vi "User Process Test.vi"() -> ()   [LabVIEW 2021, in "State Machine tests.lvlib"]
uses:
  State Machine tests.lvlib
  module/execution/State Machine runtime.lvclass
  module/execution/parameter user data.ctl
  module/execution/result user data.ctl
panel:
  in  "stop":bool
  out "error out":errorcluster
  out "Results from processing":T1
  in  "Parameters to process":T2
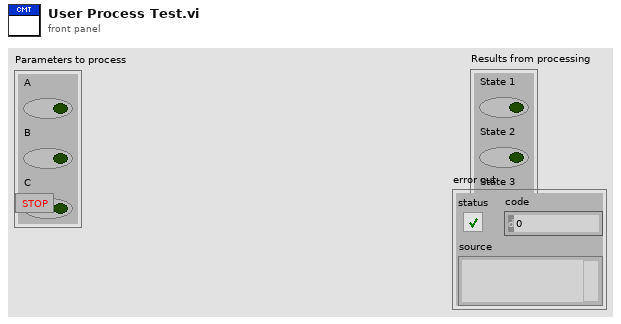
[diagram p1: front panel]
types:
  T1 = typedef "State Machine runtime.lvclass/result user data.ctl" = cluster{"State 1":bool, "State 2":bool, "State 3":bool}
  T2 = typedef "State Machine runtime.lvclass/parameter user data.ctl" = cluster{"A":bool, "B":bool, "C":bool}
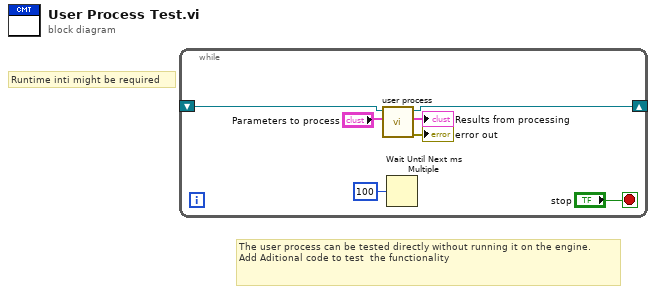
[diagram p0: block diagram]
diagram:
  # "Runtime inti might be required"
  # "The user process can be tested directly without running it on the engine.\nAdd Aditional code to test  the functionality"
  n1 = while {
    shift-right: [w1] -> _
    shift-left: _ -> [w2]
    stop <- "stop" stop-if-true
    n2 = call "user process.vi"("Parameters to process"="Parameters to process", "State Machine runtime in"=w2) -> ("error out"=→"error out":errorcluster, "Results from processing"=→"Results from processing":T1, "State Machine runtime out"=w1:refnum<class "State Machine runtime.lvclass">)  [unwired: 7 in]
    n3 = Wait Until Next ms Multiple(millisecond multiple=u32 100) -> ()  [unwired: 1 out]
  }
